vi "Clear Error (if STM closed).vi"(10 "error in":errorcluster, 11 "stm connection":T1) -> (2 "error out":errorcluster, 5 "stop?":bool)   [LabVIEW 2017, in "WinHost.lvlib"]
uses:
  WinHost.lvlib
  <vilib>/NI/STM/TCP/TCP Connection Info.ctl
  <vilib>/NI/STM/SubVIs/MetaDataElement.ctl
  <vilib>/NI/STM/NI STM.lvlib
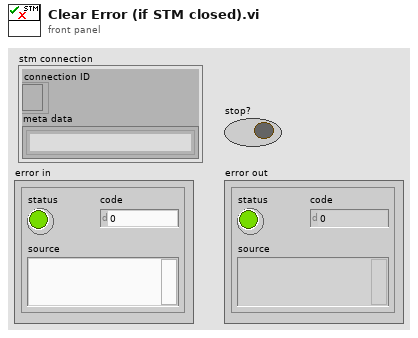
[diagram p1: front panel]
types:
  T1 = typedef "NI STM.lvlib/TCP Connection Info.ctl" = cluster{"connection ID":refnum<k5>, "meta data":T2[]}
  T2 = typedef "NI STM.lvlib/MetaDataElement.ctl" = string
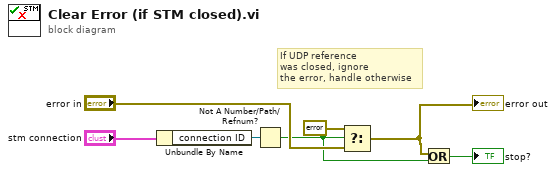
[diagram p0: block diagram]
diagram:
  # "If UDP reference\nwas closed, ignore\nthe error, handle otherwise"
  n1 = Unbundle By Name("stm connection") -> ("connection ID"=w4:refnum<k5>)
  n2 = Not A Number/Path/Refnum?(number/path/refnum=w4) -> (NaN/Path/Refnum?=w1:bool)
  n3 = Select(t=errorcluster {"status"=FALSE, "code"=0, "source"=""}, s=w1, f="error in") -> (s? t:f=w3:errorcluster)
  "error out" <- w3
  n4 = Or(x=w3, y=w1) -> (x .or. y?=→"stop?":bool)
